vi "Tag Updater.vi"() -> ()   [LabVIEW 2019]
uses:
  <vilib>/Skyline/Tag/Wrapper/Wrapper_class/Tag Value Cluster Wrapper.ctl
  <vilib>/Skyline/Configuration/Configuration_class/NI Skyline Configuration.lvclass
  <vilib>/Skyline/Tag/Shared/typedefs/Tag Value Cluster.ctl
  <vilib>/Skyline/Tag/Shared/typedefs/DataType.ctl
  <vilib>/Skyline/Utilities/Build Resource Name.vi
  <vilib>/Skyline/Tag/Wrapper/Wrapper HTTP_class/Open Tag HTTP.vi
  <vilib>/Skyline/Tag/Wrapper/Wrapper_class/Generate Tag Cluster (String) 2.vi
  <vilib>/Skyline/Tag/Wrapper/Wrapper_class/Close Tag (Single).vi
  <vilib>/Skyline/Tag/Shared/NI Skyline Tag.lvlib
  <vilib>/Skyline/Tag/Wrapper/Wrapper_class/NI Skyline Tag.lvclass
  <vilib>/Skyline/Tag/Wrapper/Wrapper HTTP_class/NI Skyline Tag HTTP.lvclass
panel:
  out "error out":errorcluster
  out "Iteration":i32
  in  "stop":bool
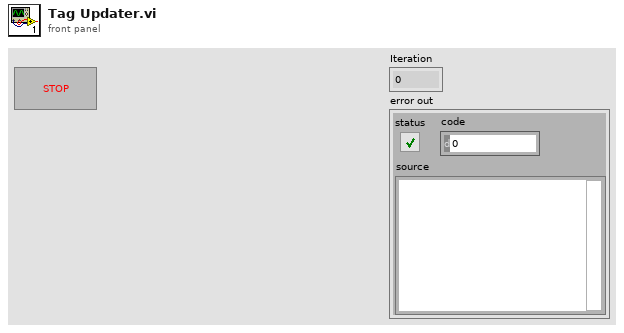
[diagram p1: front panel]
types:
  T1 = typedef "NI Skyline Tag.lvlib/DataType.ctl" = enum32{"Double", "I32", "String", "Boolean", "U64", "Timestamp"}
  T2 = typedef "NI Skyline Tag.lvclass/Tag Value Cluster Wrapper.ctl" = cluster{"Configuration":refnum<class "NI Skyline Configuration.lvclass">, "Tag Cluster":T3}
  T3 = typedef "NI Skyline Tag.lvlib/Tag Value Cluster.ctl" = cluster{"Path":string, "Data Type":T1, "Value":string, "Time Stamp":timestamp}
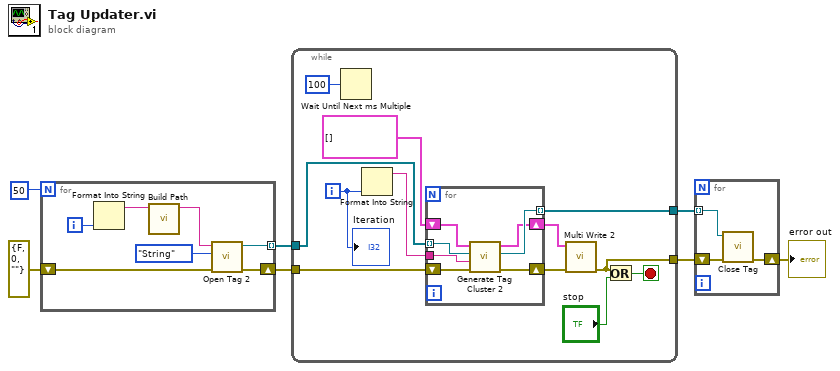
[diagram p0: block diagram]
diagram:
  n1 = for {
    N: 50 -> [_]
    tunnel: [w11] -> w6 mode=indexing
    shift-right: [w9] -> w3
    shift-left: errorcluster {"status"=FALSE, "code"=0, "source"=""} ("error out") -> [w8]
    i -> [w14]
    n2 = Format Into String(w14) -> (resulting string=w13:string)  [unwired: 3 in, 1 out]
    n3 = call <vilib>:"Build Path.vi"("tag name"=w13) -> ("path"=w12:string)  [unwired: 10 in]
    n4 = call-poly <vilib>:"Open Tag 2.vi"("error in (no error)"=w8, "Data Type"=DataType."String", "path"=w12) -> ("error out"=w9:errorcluster, "tag"=w11:refnum<class "NI Skyline Tag.lvclass">)  [unwired: 7 in]
  }
  n5 = while {
    tunnel: w6 -> [w23]
    tunnel: [w19] -> w5
    tunnel: [w17] -> w4
    tunnel: w3 -> [w22]
    i -> [w25]
    stop <- w20 stop-if-true
    n6 = Wait Until Next ms Multiple(millisecond multiple=u32 100) -> ()  [unwired: 1 out]
    n7 = Format Into String(w25) -> (resulting string=w24:string)  [unwired: 3 in, 1 out]
    n8 = for {
      tunnel: w24 -> [w33]
      tunnel: w23 -> [w32] mode=indexing
      tunnel: [w31] -> w19 mode=indexing
      shift-right: [w30] -> w18
      shift-left: w22 -> [w29]
      shift-right: [w28] -> w16
      shift-left: T2[] [] ("tag clusters out") -> [w27]
      n9 = call-poly <vilib>:"Generate Tag Cluster 2.vi"("error in (no error)"=w29, "value"=w33, "tag in"=w32, "tag clusters in"=w27) -> ("error out"=w30:errorcluster, "tag out"=w31:refnum<class "NI Skyline Tag.lvclass">, "tag clusters out"=w28:T2[])  [unwired: 5 in]
    }
    n10 = call <vilib>:"Multi Write 2.vi"("error in (no error)"=w18, "tag clusters"=w16) -> ("error out"=w17:errorcluster)  [unwired: 9 in]
    n11 = Or(x=w17, y="stop") -> (x .or. y?=w20:bool)
    "Iteration" <- w25
  }
  n12 = for {
    tunnel: w5 -> [w36] mode=indexing
    shift-right: [w34] -> w1
    shift-left: w4 -> [w35]
    n13 = call-poly <vilib>:"Close Tag.vi"("error in (no error)"=w35, "tag"=w36) -> ("error out"=w34:errorcluster)  [unwired: 9 in]
  }
  "error out" <- w1
